vi "poly_unpack_controls_cluster.vi"(2 "recursivelly? (T)":bool=TRUE, 7 "ctrl ref":refnum<vi>) -> (8 "ctrls in cluster":refnum<vi>[](array[refnum]))   [LabVIEW 2015]
uses:
  poly_is_specific_control_Cluster.vi
  cores/core_is_specific_controll.vi
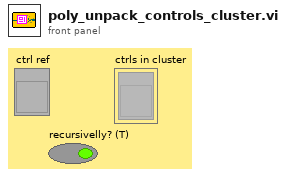
[diagram p1: front panel]
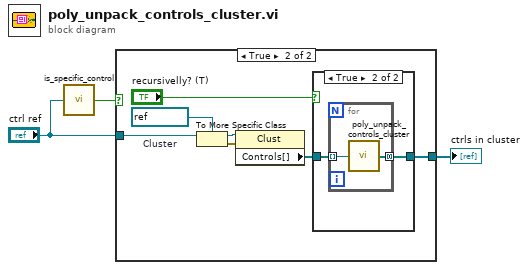
[diagram p0: block diagram]
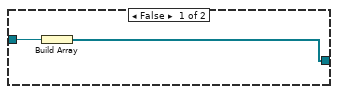
[diagram p2: hidden frame]
diagram:
  n1 = call-poly "is_specific_control.vi"("ctrl ref"="ctrl ref") -> ("is cluster?"=w1:bool)  [unwired: 8 in]
  n2 = case shown="True" w1 {
    tunnel: [w4 w7] -> w3
    tunnel: "ctrl ref" -> [w5 w9]
    frame False {
      n3 = Build Array(w5) -> (w4:refnum<vi>[])
    }
    frame True {
      w12 = refnum<vi> refnum  # Cluster
      n4 = To More Specific Class(target class=w12, reference=w9) -> (specific class reference=w10:refnum<vi>, error out=w11:errorcluster)  [unwired: 1 in]
      n5 = property class="Clust"(reference=w10, error in=w11) -> ("Controls[]"=w8:refnum<vi>[])  [unwired: 2 out]
      n6 = case shown="True" "recursivelly? (T)" {
        tunnel: w8 -> [w13 w15]
        tunnel: [w13 w14] -> w7
        frame False {
        }
        frame True {
          n7 = for {
            tunnel: w15 -> [w16] mode=indexing
            tunnel: [w17] -> w14 mode=concatenating
            n8 = call "poly_unpack_controls_cluster.vi"("ctrl ref"=w16) -> ("ctrls in cluster"=w17:refnum<vi>[])  [unwired: 14 in]
          }
        }
      }
    }
  }
  "ctrls in cluster" <- w3
